vi "AlterHeader.vi"(2 "Header In":T1={"header info"={"Header"="", "Head length"=0}, "A/D info"={"# rf points per line"=0, "# lines per scan"=0, "sample rate MHz"=0, "# A/D bits"=0, "# bytes per A/D"=0, "TGC Flag"=0, "A/D Type"=""}, "Tranducer Info"={"bandwidth"=0.0, "center freq"=0.0, "start freq"=0.0, "ID"=0}, "Scan Info"={"delay"=0.0, "pivot distance"=0.0, "sector scan angle"=0.0, "operator"="", "Scan Mode"="", "location"=""}, "Time/Date Info"={"date"="", "time"=""}, "RF Info"={"RF file name"="", "RF file att"="", "RF cal file name"="", "RF cal file att"=""}, "Patient Info"={"ID"="test", "extended ID"="", "age"=0, "sex"="", "previously\nscanned"="N", "PSA"=0.0, "LOS"=1, "Ethnicty 2"=1, "Race"=4}, "Tissue Type"={"organ"=0, "disease type"=0, "disease location"=0, "IQ_pts"=0, "RcvBuffer"=0, "RcvFrame"=0, "IQBuff"=0, "IQFrame"=0, "IQPage"=0}, "Votage scaling"={"Digitizer (dB)"=0.0, "Gain (dB)"=0.0, "Atten (dB)"=0.0}, "Comment"="", "Misc Items"={"avg num"=0, "c speed"=0, "DivideBy"=0, "XMIT CHS"=0, "RCV CHS"=0, "Tx angle"=0}, "Therapy Parameters"={"Theraputic Freq (MHz)"=0.0, "Time on (s)"=0.0, "Therapy amplitude (mV)"=0.0, "Lines Before"=0, "Lines After"=0}, "Scan Settings"={"Energy (microJ)"=0, "Damping (In Ohm)"=0, "HP Filt(KHz) "=0, "LP Filt (MHz)"=0, "Gain (db)"=0, "prf (kHz)"=0.0, "Distance between\nscan lines (um)"=0, "Distance between\nscan planes (um)"=0, "Scan line gap (um)"=0.0, "Scan plane gap (um)"=0.0}, "Compression Parameters"={"F1 (MHz)"=0.0, "F2 (MHz)"=0.0, "% taper"=0.0, "duration"=0.0}, "Patient Info Xtra"={"First Name"="", "Last Name"="", "Notes"=""}, "Boolean1"={FALSE, FALSE, FALSE, FALSE, FALSE, FALSE, FALSE, FALSE, FALSE, FALSE, FALSE, FALSE, FALSE, FALSE, FALSE, FALSE, FALSE, FALSE, FALSE, FALSE, FALSE, FALSE}, "Boolean2"={FALSE, FALSE, FALSE, FALSE, FALSE, FALSE, FALSE, FALSE, FALSE, FALSE, FALSE, FALSE, FALSE, FALSE, FALSE, FALSE, FALSE, FALSE, FALSE, FALSE, FALSE, FALSE, FALSE, FALSE, FALSE, FALSE, FALSE, FALSE, FALSE, FALSE, FALSE, FALSE, FALSE, FALSE, FALSE}, "Boolean3"={FALSE, FALSE, FALSE, FALSE, FALSE, FALSE, FALSE, FALSE, FALSE, FALSE, FALSE, FALSE, FALSE, FALSE, FALSE, FALSE, FALSE, FALSE, FALSE, FALSE, FALSE, FALSE}} {"Compression Parameters"."% taper" min=50 max=1000 format="%.2f"; "Compression Parameters"."F2 (MHz)" format="%.3f"; "Compression Parameters"."F1 (MHz)" format="%.3f"; "Scan Settings"."prf (kHz)" format="%.2f"; "Scan Settings"."Gain (db)" items=["26", "40.0", "54.0"]; "Scan Settings"."LP Filt (MHz)" items=["20", "50", "100", "200"]; "Scan Settings"."HP Filt(KHz)" items=["1", "1000", "3000", "10000"]; "Scan Settings"."Damping (In Ohm)" items=["7", "10", "16", "20", "26", "30", "40", "50"]; "Scan Settings"."Energy (microJ)" items=["1", "2", "4", "8", "16", "32"]; "Therapy Parameters"."Therapy amplitude (mV)" min=50 max=1000 format="%.2f"; "Therapy Parameters"."Time on (s)" format="%.3f"; "Therapy Parameters"."Theraputic Freq (MHz)" format="%.3f"; "Patient Info"."Race" items=["Am Ind or Alaska", "Asian", "Hawaiian, Pac Isl", "Black or Afr Amer", "White", "more than one race", "unknown"]; "Patient Info"."Ethnicty 2" items=["Hispanic", "Non-Hispanic", "unknown"]; "Patient Info"."LOS" items=["1", "2", "3", "4", "5"]; "Patient Info"."PSA" format="%.1f"; "Scan Info"."delay" format="%.2f"; "Scan Info"."pivot distance" format="%.2f"; "Scan Info"."sector scan angle" format="%.2f"; "Tranducer Info"."bandwidth" format="%.2f"; "Tranducer Info"."center freq" format="%.2f"; "Tranducer Info"."start freq" format="%.2f"}, 3 "Choose Directory":path) -> ()   [LabVIEW 2022 SP3]
panel:
  in  "Use Selected Files":bool
  in  "Listbox":i32[](listbox)
  # "Enter field to change and check box next to field. Run program,\nchoose a directory, choose the files that need their header altered, and then push \"Use Selected Files\" button."
  # "© 2000 Riverside Research Institute"
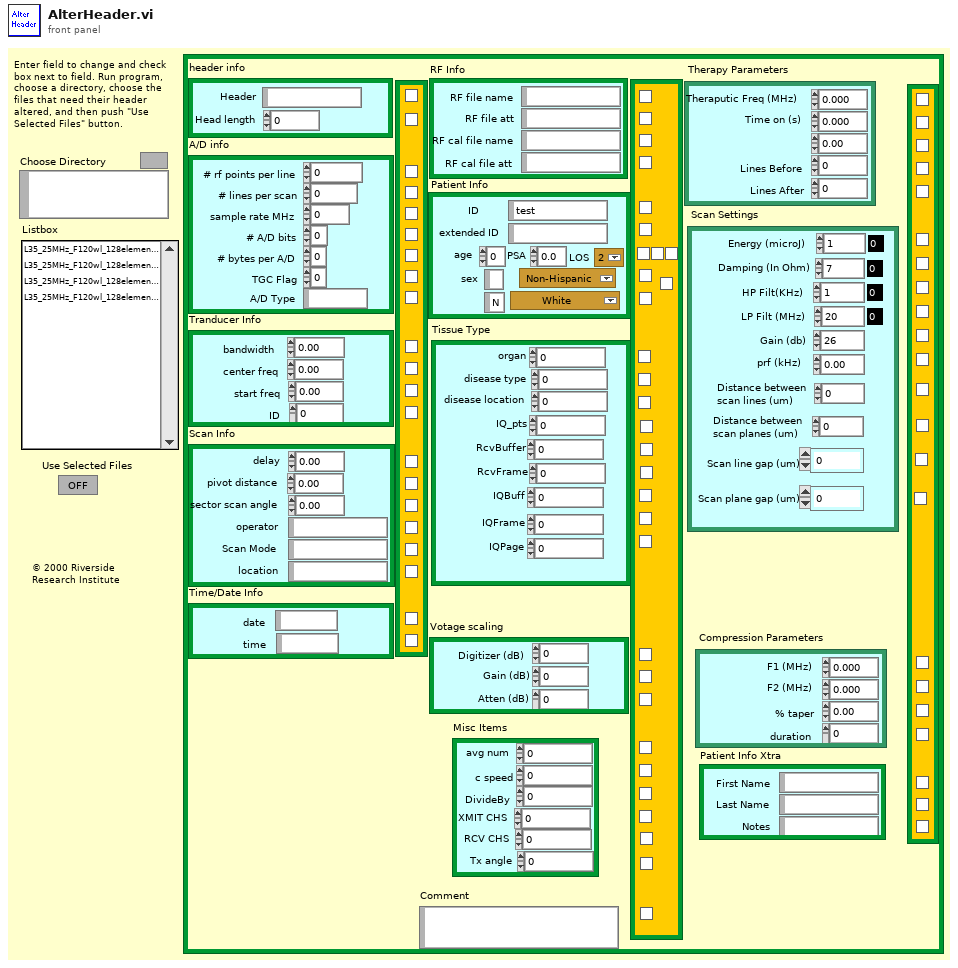
[diagram p1: front panel]
types:
  T1 = cluster{"header info":cluster{"Header":string, "Head length":i16}, "A/D info":cluster{"# rf points per line":u16, "# lines per scan":u16, "sample rate MHz":u16, "# A/D bits":i16, "# bytes per A/D":u16, "TGC Flag":u16, "A/D Type":string}, "Tranducer Info":cluster{"bandwidth":sgl, "center freq":sgl, "start freq":sgl, "ID":i32}, "Scan Info":cluster{"delay":sgl, "pivot distance":sgl, "sector scan angle":sgl, "operator":string, "Scan Mode":string, "location":string}, "Time/Date Info":cluster{"date":string, "time":string}, "RF Info":cluster{"RF file name":string, "RF file att":string, "RF cal file name":string, "RF cal file att":string}, "Patient Info":cluster{"ID":string, "extended ID":string, "age":u16, "sex":string, "previously\nscanned":string, "PSA":sgl, "LOS":u8, "Ethnicty 2":u8, "Race":u8}, "Tissue Type":cluster{"organ":i16, "disease type":i16, "disease location":i16, "IQ_pts":u16, "RcvBuffer":u8, "RcvFrame":i16, "IQBuff":u8, "IQFrame":u16, "IQPage":u8}, "Votage scaling":cluster{"Digitizer (dB)":sgl, "Gain (dB)":sgl, "Atten (dB)":sgl}, "Comment":string, "Misc Items":cluster{"avg num":i16, "c speed":i16, "DivideBy":i16, "XMIT CHS":u8, "RCV CHS":u8, "Tx angle":u8}, "Therapy Parameters":cluster{"Theraputic Freq (MHz)":sgl, "Time on (s)":sgl, "Therapy amplitude (mV)":sgl, "Lines Before":u16, "Lines After":u16}, "Scan Settings":cluster{"Energy (microJ)":u8, "Damping (In Ohm)":u8, "HP Filt(KHz) ":u8, "LP Filt (MHz)":u8, "Gain (db)":u8, "prf (kHz)":sgl, "Distance between\nscan lines (um)":u16, "Distance between\nscan planes (um)":u16, "Scan line gap (um)":sgl, "Scan plane gap (um)":sgl}, "Compression Parameters":cluster{"F1 (MHz)":sgl, "F2 (MHz)":sgl, "% taper":sgl, "duration":sgl}, "Patient Info Xtra":cluster{"First Name":string, "Last Name":string, "Notes":string}, "Boolean1":cluster{bool, bool, bool, bool, bool, bool, bool, bool, bool, bool, bool, bool, bool, bool, bool, bool, bool, bool, bool, bool, bool, bool}, "Boolean2":cluster{bool, bool, bool, bool, bool, bool, bool, bool, bool, bool, bool, bool, bool, bool, bool, bool, bool, bool, bool, bool, bool, bool, bool, bool, bool, bool, bool, bool, bool, bool, bool, bool, bool, bool, bool}, "Boolean3":cluster{bool, bool, bool, bool, bool, bool, bool, bool, bool, bool, bool, bool, bool, bool, bool, bool, bool, bool, bool, bool, bool, bool}}
  T2 = cluster{"# rf points per line":u16, "# lines per scan":u16, "sample rate MHz":u16, "# A/D bits":i16, "# bytes per A/D":u16, "TGC Flag":u16, "A/D Type":string}
  T3 = cluster{"bandwidth":sgl, "center freq":sgl, "start freq":sgl, "ID":i32}
  T4 = cluster{"delay":sgl, "pivot distance":sgl, "sector scan angle":sgl, "operator":string, "Scan Mode":string, "location":string}
  T5 = cluster{"RF file name":string, "RF file att":string, "RF cal file name":string, "RF cal file att":string}
  T6 = cluster{"ID":string, "extended ID":string, "age":u16, "sex":string, "previously\nscanned":string, "PSA":sgl, "LOS":u8, "Ethnicty 2":u8, "Race":u8}
  T7 = cluster{"organ":i16, "disease type":i16, "disease location":i16, "IQ_pts":u16, "RcvBuffer":u8, "RcvFrame":i16, "IQBuff":u8, "IQFrame":u16, "IQPage":u8}
  T8 = cluster{"Digitizer (dB)":sgl, "Gain (dB)":sgl, "Atten (dB)":sgl}
  T9 = cluster{"avg num":i16, "c speed":i16, "DivideBy":i16, "XMIT CHS":u8, "RCV CHS":u8, "Tx angle":u8}
  T10 = cluster{"Theraputic Freq (MHz)":sgl, "Time on (s)":sgl, "Therapy amplitude (mV)":sgl, "Lines Before":u16, "Lines After":u16}
  T11 = cluster{"Energy (microJ)":u8, "Damping (In Ohm)":u8, "HP Filt(KHz) ":u8, "LP Filt (MHz)":u8, "Gain (db)":u8, "prf (kHz)":sgl, "Distance between\nscan lines (um)":u16, "Distance between\nscan planes (um)":u16, "Scan line gap (um)":sgl, "Scan plane gap (um)":sgl}
  T12 = cluster{"F1 (MHz)":sgl, "F2 (MHz)":sgl, "% taper":sgl, "duration":sgl}
  T13 = cluster{"First Name":string, "Last Name":string, "Notes":string}
  T14 = cluster{bool, bool, bool, bool, bool, bool, bool, bool, bool, bool, bool, bool, bool, bool, bool, bool, bool, bool, bool, bool, bool, bool}
  T15 = cluster{bool, bool, bool, bool, bool, bool, bool, bool, bool, bool, bool, bool, bool, bool, bool, bool, bool, bool, bool, bool, bool, bool, bool, bool, bool, bool, bool, bool, bool, bool, bool, bool, bool, bool, bool}
  T16 = cluster{"header info":cluster{"Header":string, "Head length":i16}, "A/D info":cluster{"# rf points per line":u16, "# lines per scan":u16, "sample rate MHz":u16, "# A/D bits":i16, "# bytes per A/D":u16, "TGC Flag":u16, "A/D Type":string}, "Tranducer Info":cluster{"bandwidth":sgl, "center freq":sgl, "start freq":sgl, "ID":i32}, "Scan Info":cluster{"delay":sgl, "pivot distance":sgl, "sector scan angle":sgl, "operator":string, "Scan Mode":string, "location":string}, "Time/Date Info":cluster{"date":string, "time":string}, "RF Info":cluster{"RF file name":string, "RF file att":string, "RF cal file name":string, "RF cal file att":string}, "Patient Info":cluster{"ID":string, "extended ID":string, "age":u16, "sex":string, "previously\nscanned":string, "PSA":sgl, "LOS":u8, "Ethnicty 2":u8, "Race":u8}, "Tissue Type":cluster{"organ":i16, "disease type":i16, "disease location":i16, "IQ_pts":u16, "RcvBuffer":u8, "RcvFrame":i16, "IQBuff":u8, "IQFrame":u16, "IQPage":u8}, "Votage scaling":cluster{"Digitizer (dB)":sgl, "Gain (dB)":sgl, "Atten (dB)":sgl}, "Comment":string, "Misc Items":cluster{"avg num":i16, "c speed":i16, "DivideBy":i16, "XMIT CHS":u8, "RCV CHS":u8, "Tx angle":u8}, "Therapy Parameters":cluster{"Theraputic Freq (MHz)":sgl, "Time on (s)":sgl, "Therapy amplitude (mV)":sgl, "Lines Before":u16, "Lines After":u16}, "Scan Settings":cluster{"Energy (microJ)":u8, "Damping (In Ohm)":u8, "HP Filt(KHz) ":u8, "LP Filt (MHz)":u8, "Gain (db)":u8, "prf (kHz)":sgl, "Distance between\nscan lines (um)":u16, "Distance between\nscan planes (um)":u16, "Scan line gap (um)":sgl, "Scan plane gap (um)":sgl}, "Compression Parameters":cluster{"F1 (MHz)":sgl, "F2 (MHz)":sgl, "% taper":sgl, "duration":sgl}, "Patient Info Xtra":cluster{"First Name":string, "Last Name":string, "Notes":string}, "ROI Box":u16[]}
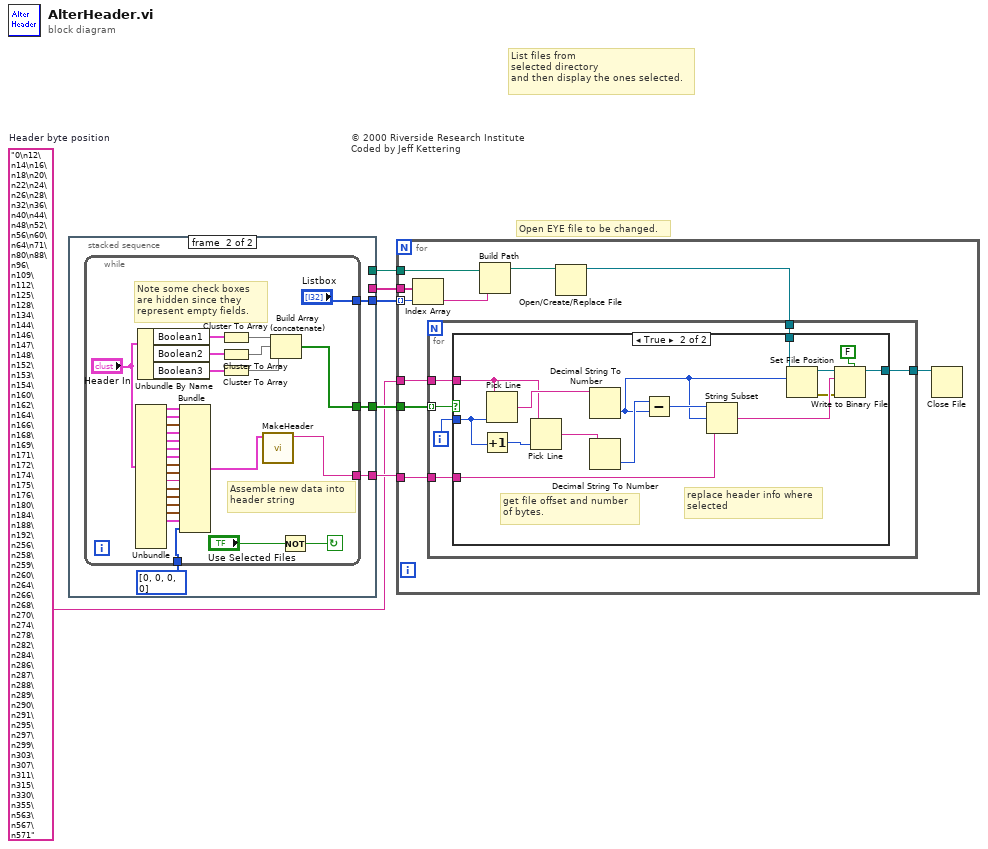
[diagram p0: block diagram]
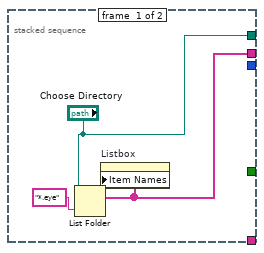
[diagram p2: hidden frame]
diagram:
  w3 = "0\n12\n14\n16\n18\n20\n22\n24\n26\n28\n32\n36\n40\n44\n48\n52\n56\n60\n64\n71\n80\n88\n96\n109\n112\n125\n128\n134\n144\n146\n147\n148\n152\n153\n154\n160\n162\n164\n166\n168\n169\n171\n172\n174\n175\n176\n180\n184\n188\n192\n256\n258\n259\n260\n264\n266\n268\n270\n274\n278\n282\n284\n286\n287\n288\n289\n290\n291\n295\n297\n299\n303\n307\n311\n315\n330\n355\n563\n567\n571"  # Header byte position
  # "© 2000 Riverside Research Institute\nCoded by Jeff Kettering"
  # "Open EYE file to be changed."
  # "List files from\nselected directory\nand then display the ones selected."
  n1 = stacked-sequence {
    tunnel: [_ w13] -> w6
    tunnel: [_ w12] -> w5
    tunnel: [_ w11] -> w4
    tunnel: [w8 _] -> w2
    tunnel: ["Choose Directory" _] -> w1
    frame #0 {
      n2 = List Folder(path="Choose Directory", pattern="*.eye") -> (filenames=w8:string[])  [unwired: 1 in, 4 out]
      n3 = property on="Listbox" class="LstBox (strict)"("Item Names"=w8) -> ()  [unwired: 2 in, 2 out]
    }
    frame #1 {
      n4 = while {
        tunnel: [w23] -> w11
        tunnel: [w24] -> w12
        tunnel: ["Listbox"] -> w13
        tunnel: u16[] [0, 0, 0, 0] ("ROI Box") -> [w15]
        stop <- w41 continue-if-true
        # "Note some check boxes\nare hidden since they represent empty fields."
        # "Assemble new data into\nheader string"
        n5 = Unbundle("Header In") -> ("header info"=w29:cluster{"Header":string, "Head length":i16}, "A/D info"=w30:T2, "Tranducer Info"=w31:T3, "Scan Info"=w32:T4, "Time/Date Info"=w33:cluster{"date":string, "time":string}, "RF Info"=w34:T5, "Patient Info"=w35:T6, "Tissue Type"=w36:T7, "Votage scaling"=w37:T8, "Comment"=w38:string, "Misc Items"=w39:T9, "Therapy Parameters"=w21:T10, "Scan Settings"=w20:T11, "Compression Parameters"=w17:T12, "Patient Info Xtra"=w16:T13)  [unwired: 3 out]
        n6 = Unbundle By Name("Header In") -> ("Boolean1"=w25:T14, "Boolean2"=w26:T15, "Boolean3"=w19:T14)
        n7 = Bundle("header info"=w29, "A/D info"=w30, "Tranducer Info"=w31, "Scan Info"=w32, "Time/Date Info"=w33, "RF Info"=w34, "Patient Info"=w35, "Tissue Type"=w36, "Votage scaling"=w37, "Comment"=w38, "Misc Items"=w39, "Therapy Parameters"=w21, "Scan Settings"=w20, "Compression Parameters"=w17, "Patient Info Xtra"=w16, "ROI Box"=w15) -> (w14:T16)  [unwired: 1 out]
        n8 = Cluster To Array(cluster=w25) -> (array=w27:bool[])
        n9 = Cluster To Array(cluster=w26) -> (array=w28:bool[])
        n10 = Cluster To Array(cluster=w19) -> (array=w18:bool[])
        n11 = call "MakeHeader.vi"("Header In"=w14) -> ("Header String"=w23:string)  [unwired: 6 out]
        n12 = Build Array (concatenate)(w27, w28, w18) -> (w24:bool[])
        n13 = Not(x="Use Selected Files") -> (.not. x?=w41:bool)
      }
    }
  }
  n14 = for {
    tunnel: w6 -> [w52] mode=indexing
    tunnel: w2 -> [w51]
    tunnel: w4 -> [w44]
    tunnel: w5 -> [w49]
    tunnel: w3 -> [w48]
    tunnel: w1 -> [w43]
    n15 = Index Array(array=w51, index=w52) -> (element=w50:string)
    n16 = Build Path(base path=w43, name or relative path=w50) -> (appended path=w47:path)
    n17 = Open/Create/Replace File(file path (use dialog)=w47) -> (refnum out=w46:refnum<file>)  [unwired: 1 in, 6 out]
    n18 = for {
      tunnel: w49 -> [w58] mode=indexing
      tunnel: w48 -> [w57]
      tunnel: w46 -> [w55]
      tunnel: [w54] -> w45
      tunnel: w44 -> [w53]
      i -> [w56]
      n19 = case shown="True" w58 {
        tunnel: w57 -> [_ w66]
        tunnel: w56 -> [_ w74]
        tunnel: w55 -> [w59 w68]
        tunnel: [w59 w67] -> w54
        tunnel: w53 -> [_ w65]
        frame False {
        }
        frame True {
          # "get file offset and number\nof bytes."
          # "replace header info where\nselected"
          n20 = Increment(x=w74) -> (x+1=w73:i32)
          n21 = Pick Line(multi-line string=w66, line index=w74) -> (output string=w72:string)  [unwired: 1 out]
          n22 = Pick Line(multi-line string=w66, line index=w73) -> (output string=w71:string)  [unwired: 1 out]
          n23 = Decimal String To Number(string=w72) -> (number=w63:i32)  [unwired: 3 out]
          n24 = Decimal String To Number(string=w71) -> (number=w64:i32)  [unwired: 3 out]
          n25 = Subtract(x=w64, y=w63) -> (x-y=w70:i32)
          n26 = String Subset(string=w65, offset (0)=w63, length (rest)=w70) -> (substring=w69:string)
          n27 = Set File Position(offset (in bytes) (0)=w63, refnum=w68) -> (refnum out=w62:refnum<file>, error out=w61:errorcluster)  [unwired: 1 in, 1 out]
          n28 = Write to Binary File(file (use dialog)=w62, data=w69, error in=w61, 5:FALSE ("prepend array or string size? (T)")) -> (refnum out=w67:refnum<file>)  [unwired: 4 out]
        }
      }
    }
    n29 = Close File(refnum=w45) -> ()  [unwired: 1 in, 2 out]
  }
